vi "GlobalPrevPage.vi"() -> ()   [LabVIEW 2013]
panel:
  in  "Prev Data Page":dbl
  in  "Prev Param Page":dbl
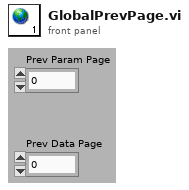
[diagram p1: front panel]
diagram:
